vi "Create Default Attributes.vi"(5 "Unique ID":string, 7 "Process Executive Ref":refnum<data-value>, 11 "Stop Air Dry in":refnum<class "Stop Air Dry.lvclass">) -> (3 "Stop Air Dry out":refnum<class "Stop Air Dry.lvclass">)   [LabVIEW 2019, in "Stop Air Dry.lvclass"]
uses:
  <vilib>/gpm_packages/@cs/Car-wash/Source/Process Steps/Stop Air Dry/Stop Air Dry.lvclass
  <vilib>/gpm_packages/@cs/test-executive/Source/Test Executive/ITestExecutive/ITest Executive.lvclass
  a30d43d8-38a5-4371-88e2-5bd4b4cee778.vi
  <vilib>/Utility/error.llb/Error Cluster From Error Code.vi
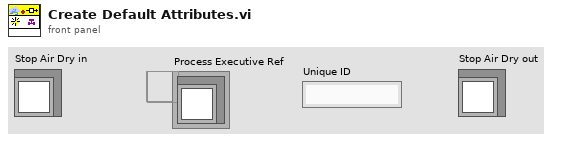
[diagram p1: front panel]
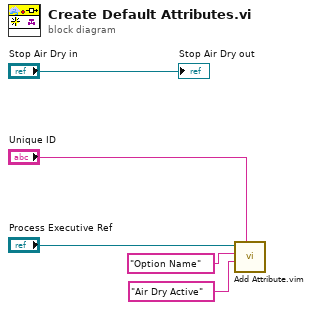
[diagram p0: block diagram]
diagram:
  n1 = call "Add Attribute.vim"("ID"="Unique ID", "Attribute"="Air Dry Active" ("Item Name"), "Attribute Name"="Option Name" ("Item Name"), "Test Executive Ref"="Process Executive Ref") -> ()  [unwired: 4 in, 4 out]
  "Stop Air Dry out" <- "Stop Air Dry in"
